vi "PH_O2_Watch.contents.vi"   [LabVIEW 2014, in "PH_O2_Watch.lvlib"]
doc: "This class is forseen read out the value of an oxid sensor. \n\nThis class is part of the PHELIX device layer."
uses:
  PH_O2_Watch.lvlib
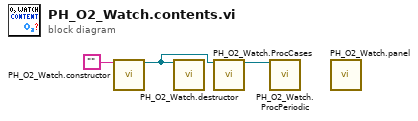
[diagram p0: block diagram]
diagram:
  n1 = call "PH_O2_Watch.constructor.vi"("name"="") -> ("i ref out"=w1:refnum<vi>)  [unwired: 16 in, 2 out]
  n2 = call "PH_O2_Watch.destructor.vi"("i ref in"=w1) -> ()  [unwired: 18 in, 1 out]
  n3 = call "PH_O2_Watch.ProcCases.vi"("i ref in"=w1) -> ("i ref out"=w3:refnum<vi>)  [unwired: 16 in, 2 out]
  n4 = call "PH_O2_Watch.ProcPeriodic.vi"("i ref in"=w3) -> ()  [unwired: 16 in, 3 out]
  n5 = call "PH_O2_Watch.panel.vi"() -> ()  [unwired: 19 in, 1 out]
